vi "Read.vi"(8 "error in (no error)":errorcluster, 9 "timeout ms (5000)":i32=5000, 11 "WebSocket in":refnum<class "WebSocket.lvclass">) -> (0 "error out":errorcluster, 1 "Opcode":T1=1 items=["Cont. Frame"=0, "Text"=1, "Binary"=2, "Ping"=9, "Pong"=10], 2 "Data":string, 3 "WebSocket out":refnum<class "WebSocket.lvclass">, 4 "Finished?":bool)   [LabVIEW 2021, in "WebSockets.lvlib"]
doc: "**Deprecated - please use the new WebSocket.lvclass VIs instead. VI is retained for backwards compatibility.**\n\nReads and decodes an incoming WebSockets message.\n\nOpcode: Opcode for the message.\nData: Contains the WebSockets payload\nFinished?: Determines whether the message is complete for fragmented messages. If false, must continue to read messages (continuation frames with opcode = 0) until Finished? is true.\nWebSockets 2.0.1.40\nSam Sharp - MediaMongrels Ltd\nCopyright (c) 2019, MediaMongrels Ltd"
uses:
  WebSockets.lvlib
  WebSocket/WebSocket.lvclass
  WebSocket/Opcodes.ctl
  WebSocket/WebSocket.lvclass/WebSocket.ctl
  Timing/Calculate Timeout.vi
  Timing/Tick Count with Error Wires.vi
  <vilib>/Utility/error.llb/Error Cluster From Error Code.vi
  WebSocket/DecodeMaskedBytes.vi
  Sockets/Socket/Socket.lvclass
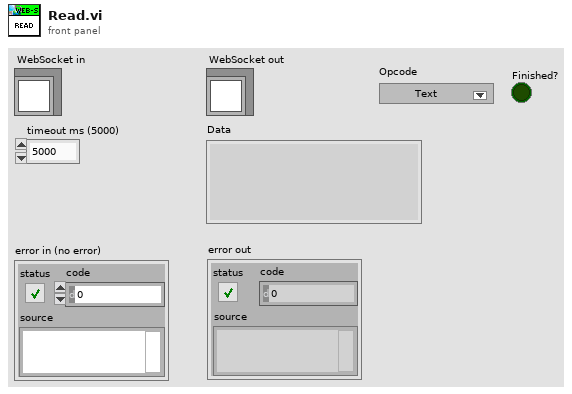
[diagram p1: front panel]
types:
  T1 = typedef "WebSockets.lvlib/WebSocket.lvclass/Opcodes.ctl" = u8
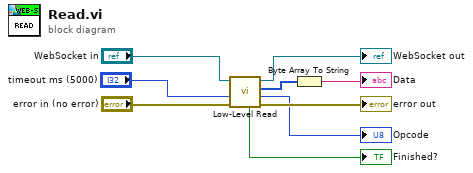
[diagram p0: block diagram]
diagram:
  n1 = call "Low-Level Read.vi"("error in (no error)"="error in (no error)", "timeout ms (5000)"="timeout ms (5000)", "WebSockets in"="WebSocket in") -> ("error out"=→"error out":errorcluster, "Opcode"=→"Opcode":T1, "Data"=w2:u8[], "WebSockets out"=→"WebSocket out":refnum<class "WebSocket.lvclass">, "Finished?"=→"Finished?":bool)  [unwired: 4 in]
  n2 = Byte Array To String(unsigned byte array=w2) -> (string=→"Data":string)
